vi "Start Button Scroll.vi"(8 "error in (no error)":errorcluster, 10 "CtlRef":refnum<vi>, 11 "SwipeMenu in":refnum<class "SwipeMenu.lvclass">) -> (0 "error out":errorcluster, 3 "SwipeMenu out":refnum<class "SwipeMenu.lvclass">)   [LabVIEW 2019, in "SwipeMenu.lvclass"]
uses:
  SwipeMenu.lvclass
  SwipeMenu.lvclass/SwipeMenu.ctl
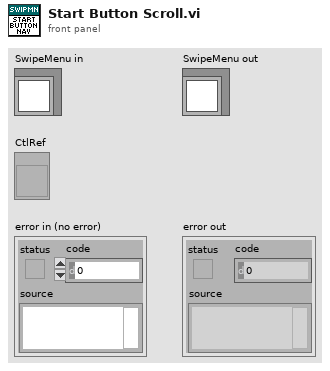
[diagram p1: front panel]
types:
  T1 = enum16{"Idle", "Mouse Nav", "Slowdown", "Button Nav"}
  T2 = typedef "SwipeMenu.lvclass/State Data.ctl" = cluster{"State":enum16{"Idle", "Mouse Nav", "Slowdown", "Button Nav"}, "Timeout":i32, "Time":timestamp, "Position":i32, "Scroll Position":i16, "Rate":dbl, "Direction":enum16{"Left", "Right"}}
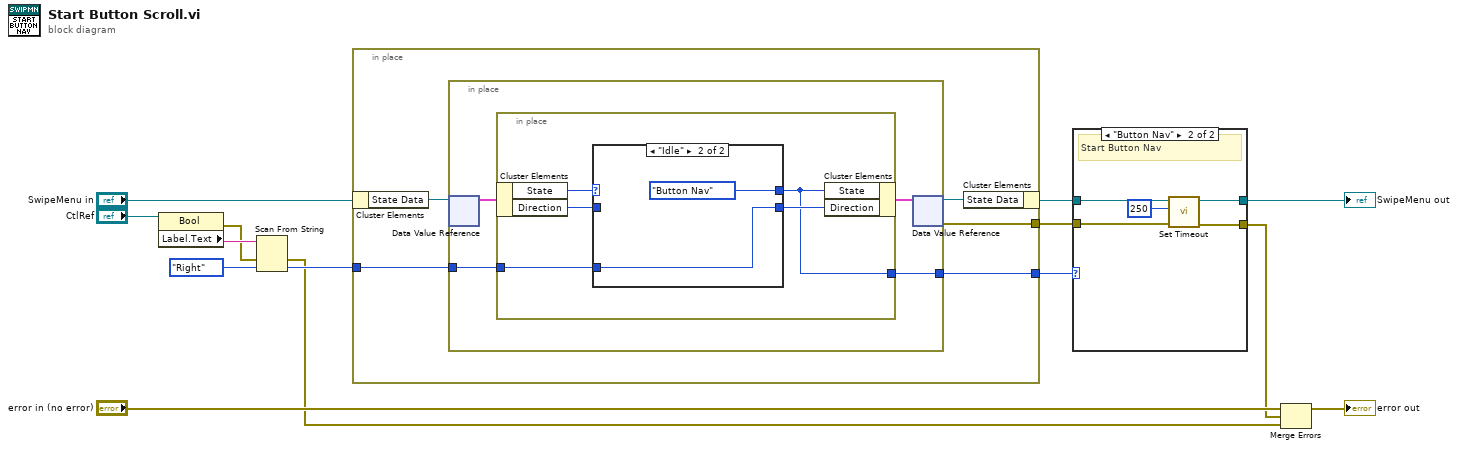
[diagram p0: block diagram]
diagram:
  n1 = property class="Bool"(reference="CtlRef") -> (error out=w2:errorcluster, "Label.Text"=w12:string)  [unwired: 1 in, 1 out]
  n2 = Scan From String(input string=w12, error in=w2, default 1=enum16{"Left", "Right"}."Right" ("Direction")) -> (error out=w1:errorcluster, output 1=w9:enum16{"Left", "Right"})  [unwired: 2 in, 2 out]
  n3 = in-place {
    in-place-border: [w17] -> w8
    in-place-border: [w16] -> w5
    in-place-border: w9 -> [w15]
    n4 = in-place-cluster #1("SwipeMenu in") -> ("State Data"=w19:refnum<data-value>)
    n5 = in-place {
      in-place-border: [w21] -> w17
      in-place-border: w15 -> [w22]
      n6 = in-place-dvr #2(w19) -> (w23:T2)  [unwired: 1 out]
      n7 = in-place {
        in-place-border: w22 -> [w25]
        in-place-border: [w24] -> w21
        n8 = in-place-cluster #3(w23) -> ("State"=w28:T1, "Direction"=w26:enum16{"Left", "Right"})
        n9 = case shown="\"Idle\"" w28 {
          selector: w28 -> [w30 _]
          tunnel: [w30 T1."Button Nav" ("State")] -> w24
          tunnel: [w29 w31] -> w27
          tunnel: w26 -> [w29 _]
          tunnel: w25 -> [_ w31]
          frame Default {
          }
          frame "Idle" {
          }
        }
        n10 = in-place-cluster #3("State"=w24, "Direction"=w27) -> (w20:T2)
      }
      n11 = in-place-dvr #2(w20) -> (w18:refnum<data-value>, w16:errorcluster)
    }
    n12 = in-place-cluster #1("State Data"=w18) -> (w7:refnum<class "SwipeMenu.lvclass">)
  }
  n13 = case shown="\"Button Nav\"" w8 {
    tunnel: w7 -> [w34 w39]
    tunnel: [w34 w37] -> w6
    tunnel: w5 -> [w33 w36]
    tunnel: [w33 w35] -> w3
    frame Default {
      # "Busy"
    }
    frame "Button Nav" {
      # "Start Button Nav"
      n14 = call "Set Timeout.vi"("error in (no error)"=w36, "Timeout"=250, "SwipeMenu in"=w39) -> ("error out"=w35:errorcluster, "SwipeMenu out"=w37:refnum<class "SwipeMenu.lvclass">)  [unwired: 7 in]
    }
  }
  "SwipeMenu out" <- w6
  n15 = Merge Errors("error in (no error)", w3, w1) -> (→"error out":errorcluster)
